vi "Get Wheel Type.vi"(8 "error in (no error)":errorcluster, 11 "fixed wheel in":refnum<class "NI_Robotics_Fixed Wheel.lvclass">) -> (0 "error out":errorcluster, 2 "Wheel Type":string, 3 "fixed wheel out":refnum<class "NI_Robotics_Fixed Wheel.lvclass">)   [LabVIEW 2017, in "NI_Robotics_Fixed Wheel.lvclass"]
uses:
  <vilib>/robotics/Steering/Fixed Wheel/NI_Robotics_Fixed Wheel.lvclass
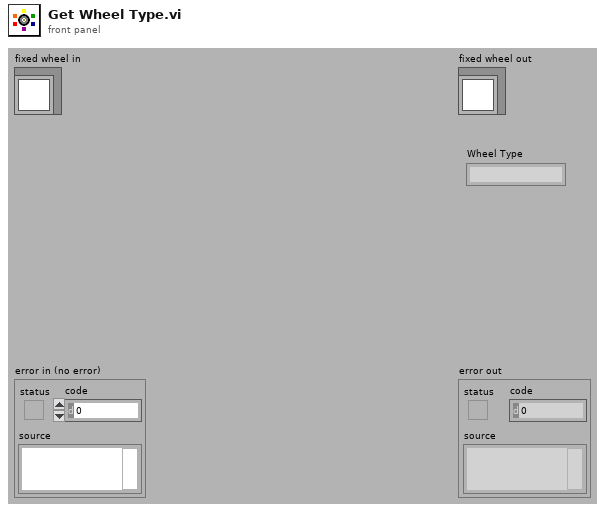
[diagram p1: front panel]
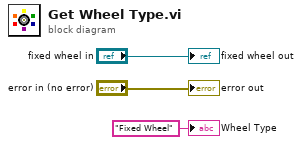
[diagram p0: block diagram]
diagram:
  "error out" <- "error in (no error)"
  "fixed wheel out" <- "fixed wheel in"
  "Wheel Type" <- "Fixed Wheel" ("Wheel Type")
